vi "Runing Fan.vi"() -> ()   [LabVIEW 2024]
panel:
  in  "stop":bool
  in  "Boolean":bool
  in  "Numeric":dbl
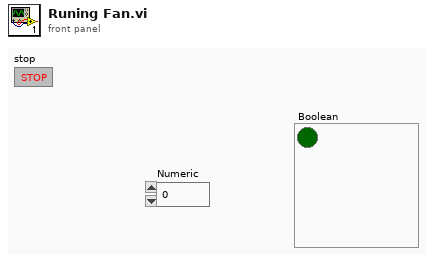
[diagram p1: front panel]
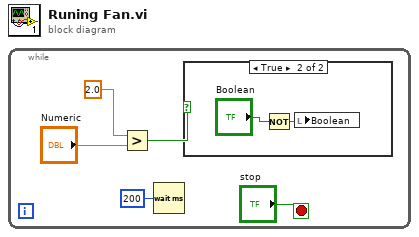
[diagram p0: block diagram]
diagram:
  n1 = while {
    stop <- "stop" stop-if-true
    n2 = Greater?(x=2.0, y="Numeric") -> (0:w1:bool)
    n3 = Wait (ms)(milliseconds to wait=u32 200 ("millisecond multiple")) -> ()  [unwired: 1 out]
    n4 = case shown="True" w1 {
      frame False {
      }
      frame True {
        n5 = Not(x="Boolean") -> (.not. x?=w6:bool)
        n6 = local write "Boolean"(w6) -> ()
      }
    }
  }
